vi "Configuration.vi"() -> (0 "firmware version":string(combo)="AH2X0208", 1 "Reset":bool, 2 "ID Query":bool=TRUE, 3 "VISA resource name out":refnum<visa-resource-name>, 5 "serial configuration out":T1={"Baud Rate"=9600, "Parity"=0, "Data Bits"=8, "Stop Bits"=10, "Flow Control"=0} {"Flow Control" items=["None", "XON/XOFF", "RTS/CTS", "XON/XOFF & RTS/CTS", "DTR/DSR", "XON/XOFF & DTR/DSR"]; "Stop Bits" items=["1.0"=10, "1.5"=15, "2.0"=20]; "Data Bits" items=["7"=7, "8"=8]; "Parity" items=["None", "Odd", "Even", "Mark", "Space"]; "Baud Rate" items=["300"=300, "600"=600, "1200"=1200, "2400"=2400, "4800"=4800, "9600"=9600, "19200"=19200]})   [LabVIEW 2021, in "Andeen-Hagerling 2700A.lvlib"]
doc: "Prompt the user for configuration parameters which can be used for initialization."
uses:
  Andeen-Hagerling 2700A.lvlib
panel:
  in  "firmware version":string(combo)="AH2X0208"
  in  "ID Query":bool=TRUE
  in  "Reset":bool=TRUE
  in  "OK Button":bool
  in  "serial configuration":T1={"Baud Rate"=9600, "Parity"=0, "Data Bits"=8, "Stop Bits"=10, "Flow Control"=0} {"Flow Control" items=["None", "XON/XOFF", "RTS/CTS", "XON/XOFF & RTS/CTS", "DTR/DSR", "XON/XOFF & DTR/DSR"]; "Stop Bits" items=["1.0"=10, "1.5"=15, "2.0"=20]; "Data Bits" items=["7"=7, "8"=8]; "Parity" items=["None", "Odd", "Even", "Mark", "Space"]; "Baud Rate" items=["300"=300, "600"=600, "1200"=1200, "2400"=2400, "4800"=4800, "9600"=9600, "19200"=19200, "38400"=38400, "57600"=57600, "115200"=115200]}
  in  "VISA resource name":refnum<visa-resource-name>="COM1"
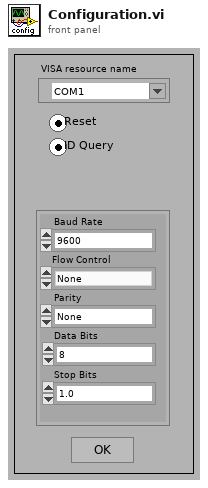
[diagram p1: front panel]
types:
  T1 = cluster{"Baud Rate":u32, "Parity":u16, "Data Bits":u16, "Stop Bits":u16, "Flow Control":u16}
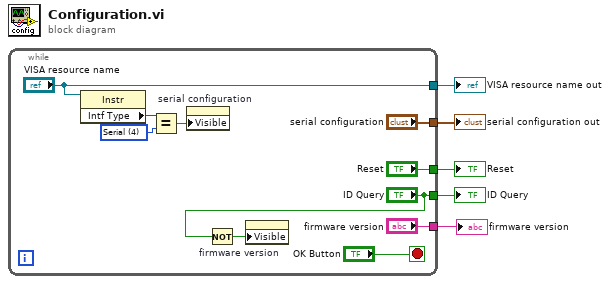
[diagram p0: block diagram]
diagram:
  n1 = while {
    tunnel: ["serial configuration"] -> w5
    tunnel: ["VISA resource name"] -> w4
    tunnel: ["Reset"] -> w3
    tunnel: ["ID Query"] -> w2
    tunnel: ["firmware version"] -> w1
    stop <- "OK Button" stop-if-true
    w11 = u16 4 items=["GPIB"=1, "VXI"=2, "GPIB-VXI"=3, "Serial"=4, "PXI"=5, "TCPIP"=6, "USB"=7, "FireWire"=9] ("Interface Information:Interface Type")
    n2 = property class="Instr"(reference="VISA resource name") -> ("Intf Type"=w12:u16)  [unwired: 1 in, 2 out]
    n3 = Equal?(x=w12, y=w11) -> (x = y?=w10:bool)
    n4 = property on="serial configuration" class="Clust (strict)"("Visible"=w10) -> ()  [unwired: 2 in, 2 out]
    n5 = Not(x="ID Query") -> (.not. x?=w7:bool)
    n6 = property on="firmware version" class="CmbBox"("Visible"=w7) -> ()  [unwired: 2 in, 2 out]
  }
  "VISA resource name out" <- w4
  "serial configuration out" <- w5
  "Reset" <- w3
  "ID Query" <- w2
  "firmware version" <- w1
